vi "RESTful Control Type To XMLType.vi"(1 "Type Enum":T1) -> (0 "Control Type XML":string)   [LabVIEW 2020]
uses:
  <vilib>/Utility/VariantDataType/Type.ctl
  <vilib>/Utility/VariantDataType/VariantType.lvlib
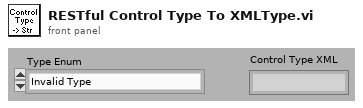
[diagram p1: front panel]
types:
  T1 = typedef "VariantType.lvlib/Type.ctl" = enum8{"Invalid Type", "Void", "I8", "I16", "I32", "I64", "U8", "U16", "U32", "U64", "Single Float", "Double Float", "Extended Float", "Single Complex", "Double Complex", "Extended Complex", "Enum U8", "Enum U16", "Enum U32", "Enum U64", "Single Float With Unit", "Double Float With Unit", "Extended Float With Unit", "Single Complex with Unit", "Double Complex with Unit", "Extended Complex with Unit", "Boolean", "String", "Path", "Picture", "Tag", "Array", "Cluster", "Variant", "LV Variant", "Waveform", "Timestamp", "Digital Waveform", "Digital Data", "ExpressData", "Refnum", "External Data", "VI", "Poly VI", "LabVIEW Class Instance", "Fixed Point"}
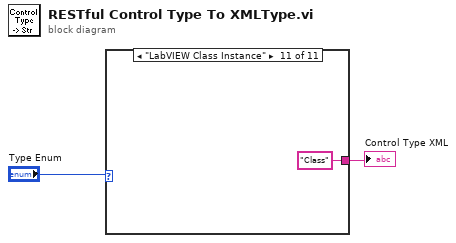
[diagram p0: block diagram]
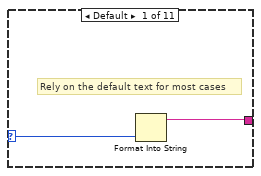
[diagram p2: hidden frame]
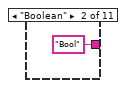
[diagram p3: hidden frame]
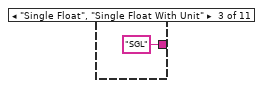
[diagram p4: hidden frame]
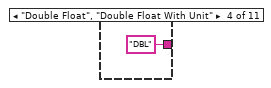
[diagram p5: hidden frame]
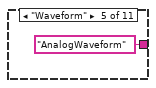
[diagram p6: hidden frame]
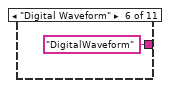
[diagram p7: hidden frame]
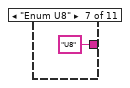
[diagram p8: hidden frame]
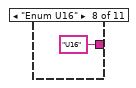
[diagram p9: hidden frame]
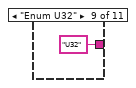
[diagram p10: hidden frame]
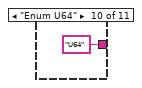
[diagram p11: hidden frame]
diagram:
  n1 = case shown="\"LabVIEW Class Instance\"" "Type Enum" {
    selector: "Type Enum" -> [w4 _ _ _ _ _ _ _ _ _ _]
    tunnel: [w3 "Bool" ("Boolean Text") "SGL" ("Boolean Text") "DBL" ("Boolean Text") "AnalogWaveform" ("Boolean Text") "DigitalWaveform" ("Boolean Text") "U8" ("Boolean Text") "U16" ("Boolean Text") "U32" ("Boolean Text") "U64" ("Boolean Text") "Class" ("Boolean Text")] -> w1
    frame Default {
      # "Rely on the default text for most cases"
      n2 = Format Into String(w4) -> (resulting string=w3:string)  [unwired: 3 in, 1 out]
    }
    frame "Boolean" {
    }
    frame "Single Float", "Single Float With Unit" {
    }
    frame "Double Float", "Double Float With Unit" {
    }
    frame "Waveform" {
    }
    frame "Digital Waveform" {
    }
    frame "Enum U8" {
    }
    frame "Enum U16" {
    }
    frame "Enum U32" {
    }
    frame "Enum U64" {
    }
    frame "LabVIEW Class Instance" {
    }
  }
  "Control Type XML" <- w1
